vi "Write RelatedIssues.vi"(8 "error in (no error)":errorcluster, 10 "RelatedIssues":dbl, 11 "Component in":refnum<class "Component.lvclass">) -> (0 "error out":errorcluster, 3 "Component out":refnum<class "Component.lvclass">)   [LabVIEW 2018, in "Component.lvclass"]
uses:
  Component.lvclass
  Component.lvclass/Component.ctl
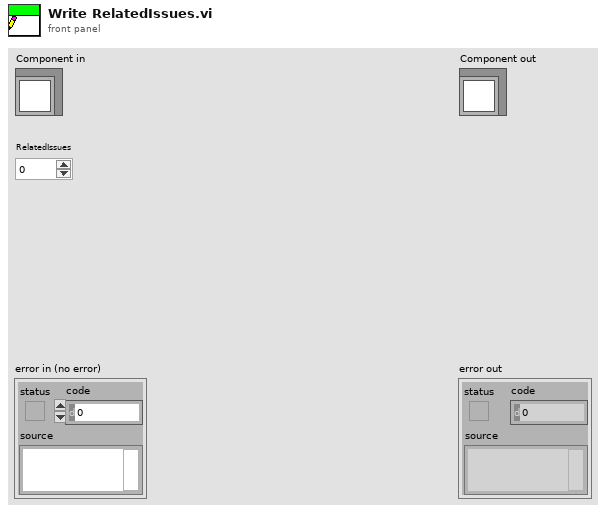
[diagram p1: front panel]
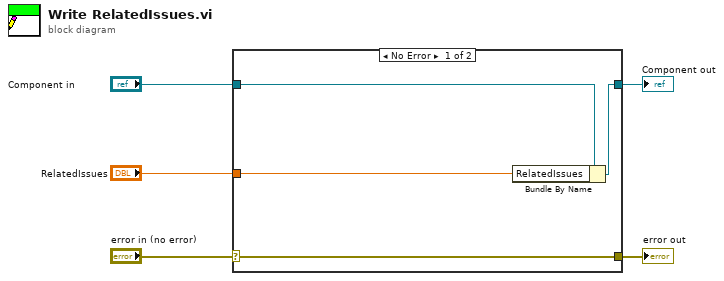
[diagram p0: block diagram]
diagram:
  n1 = case shown="No Error" "error in (no error)" {
    selector: "error in (no error)" -> [w9 w10]
    tunnel: [w9 w10] -> w4
    tunnel: [w7 w11] -> w2
    tunnel: "Component in" -> [w8 w11]
    tunnel: "RelatedIssues" -> [w6 _]
    frame No Error {
      n2 = Bundle By Name(cluster=w8, "RelatedIssues"=w6) -> (w7:refnum<class "Component.lvclass">)
    }
    frame Error {
    }
  }
  "error out" <- w4
  "Component out" <- w2
